vi "Timed Progress Bar Caller.vi"(8 "Error In":errorcluster, 10 "Delay Label":string, 11 "Time Delay in MS":i32=10) -> (0 "Error Out":errorcluster)   [LabVIEW 2018]
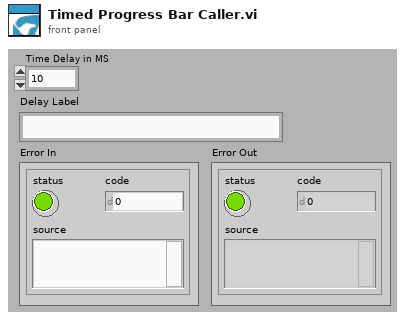
[diagram p1: front panel]
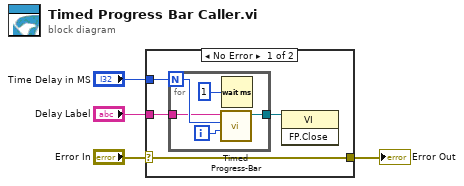
[diagram p0: block diagram]
diagram:
  n1 = case shown="No Error" "Error In" {
    selector: "Error In" -> [w7 w14]
    tunnel: [w7 w14] -> w3
    tunnel: "Time Delay in MS" -> [w6 _]
    tunnel: "Delay Label" -> [w5 _]
    frame No Error {
      n2 = for {
        N: w6 -> [w11]
        tunnel: [w12] -> w8
        tunnel: w5 -> [w9]
        i -> [w10]
        n3 = call "Timed Progress-Bar.vi"("Delay Label"=w9, "Size"=w11, "Increment"=w10) -> ("Prog Bar Ref"=w12:refnum<vi>)  [unwired: 6 in]
        n4 = Wait (ms)(milliseconds to wait=u32 1) -> ()  [unwired: 1 out]
      }
      n5 = invoke class="VI" method="FP.Close"(reference=w8) -> ()  [unwired: 2 in, 3 out]
    }
    frame Error {
    }
  }
  "Error Out" <- w3
